vi "Frame create.vi"(7 "Command":string, 8 "error in (no error)":errorcluster, 11 "ISO 14443 A UP in":refnum<class "ISO 14443 A UP.lvclass">) -> (0 "error out":errorcluster, 3 "ISO 14443 A UP out":refnum<class "ISO 14443 A UP.lvclass">)   [LabVIEW 2019, in "ISO 14443 A UP.lvclass"]
uses:
  ISO 14443 A UP.lvclass
  TypeDef/Store.ctl
  ISO 14443 A UP.lvclass/ISO 14443 A UP.ctl
  RFID system.lvclass
panel:
  in  "LSB":u8[](array[numeric])=[80] format="%x"
  in  "MSB":u8[](array[numeric])=[178] format="%x"
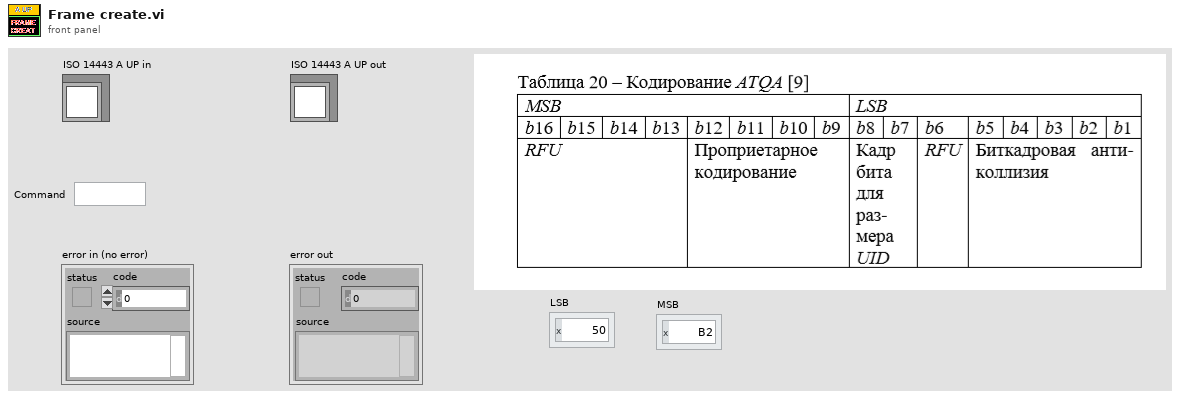
[diagram p1: front panel]
types:
  T1 = typedef "Store.ctl" = enum16{"envelope", "noise", "demSubCar", "CH_frame", "Decode", "demodulate", "in", "out", "sum", "subCarrier", "frame", "command", "encode", "modulate", "encode_UP", "modulate_up", "demod_up", "envelop_up", "sum_up", "out_up", "in_up"}
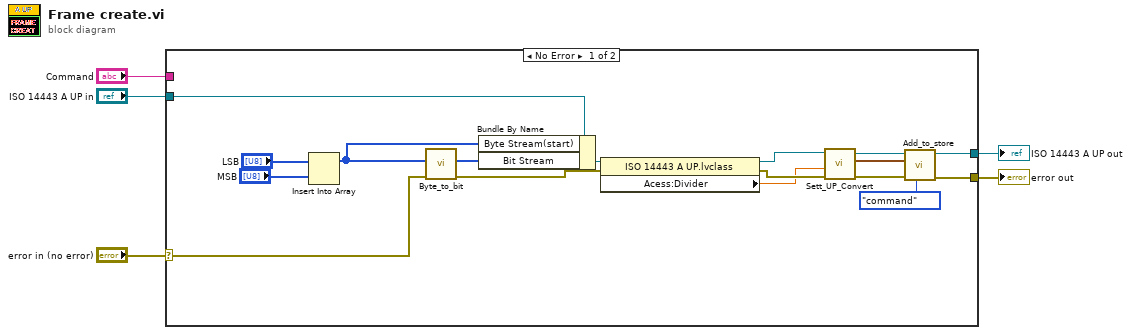
[diagram p0: block diagram]
diagram:
  n1 = case shown="No Error" "error in (no error)" {
    selector: "error in (no error)" -> [w19 w23]
    tunnel: [w11 w23] -> w4
    tunnel: "ISO 14443 A UP in" -> [w18 w24]
    tunnel: [w14 w24] -> w2
    tunnel: "Command" -> [_ _]
    frame No Error {
      n2 = Insert Into Array(array="LSB", new element="MSB") -> (w20:u8[])  [unwired: 1 in]
      n3 = call "Byte_to_bit.vi"("Error In"=w19, "Array of byte"=w20) -> ("Error Out"=w8:errorcluster, "Arrray of bit"=w17:u8[])  [unwired: 5 in, 1 out]
      n4 = Bundle By Name(cluster=w18, "Byte Stream(start)"=w20, "Bit Stream"=w17) -> (w16:refnum<class "ISO 14443 A UP.lvclass">)
      n5 = property class="ISO 14443 A UP.lvclass"(reference=w16, error in=w8) -> (reference out=w9:refnum<class "ISO 14443 A UP.lvclass">, error out=w7:errorcluster, "Acess:Divider"=w6:dbl)
      n6 = call-dynamic "Sett_UP_Convert.vi"("error in (no error)"=w7, "Divider(1)"=w6, "ISO 14443 A UP in"=w9) -> ("error out"=w13:errorcluster, "Waveform"=w12:waveform(dbl), "ISO 14443 A UP out"=w15:refnum<class "ISO 14443 A UP.lvclass">)  [unwired: 6 in]
      n7 = call "Add_to_store.vi"("Store"=Store."command", "error in (no error)"=w13, "Waveform"=w12, "RFID system in"=w15) -> ("error out"=w11:errorcluster, "RFID system out"=w14:refnum<class "ISO 14443 A UP.lvclass">)  [unwired: 6 in]
    }
    frame Error {
    }
  }
  "error out" <- w4
  "ISO 14443 A UP out" <- w2
